vi "ISX3_Cmd_GetSetupSize.vi"() -> (0 "get Setup Size Cmd":u8[](array[numeric]))   [LabVIEW 2012, in "Sciospec ISX3 Impedance Analyzer.lvlib"]
uses:
  Sciospec ISX3 Impedance Analyzer.lvlib
panel:
  # "This VI generates the command to get the number of frequencies in the configured setup."
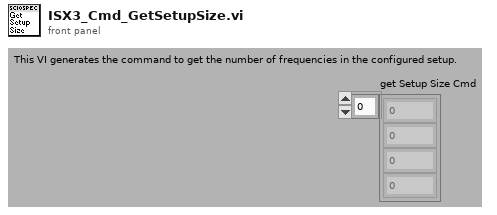
[diagram p1: front panel]
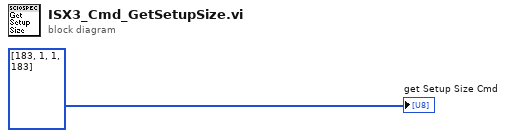
[diagram p0: block diagram]
diagram:
  "get Setup Size Cmd" <- u8[] [183, 1, 1, 183]
